vi "Update Position.vi"(11 "Motion in":refnum<class "Motion.lvclass">) -> (3 "Motion out":refnum<class "Motion.lvclass">)   [LabVIEW 2021, in "Motion.lvclass"]
uses:
  Motion.lvclass
  Motion.lvclass/Motion.ctl
  Re-use Libraries/Vector 2D/Vector 2D.lvclass
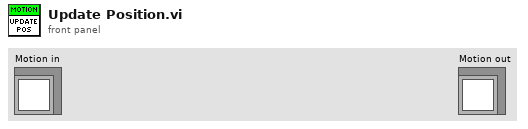
[diagram p1: front panel]
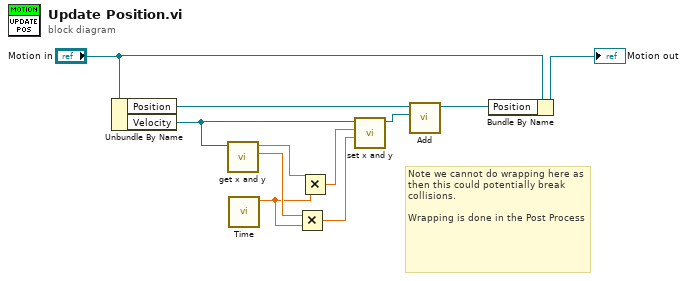
[diagram p0: block diagram]
diagram:
  # "Note we cannot do wrapping here as then this could potentially break collisions.\n\nWrapping is done in the Post Process"
  n1 = Unbundle By Name("Motion in") -> ("Position"=w11:refnum<class "Vector 2D.lvclass">, "Velocity"=w6:refnum<class "Vector 2D.lvclass">)
  n2 = call "get x and y.vi"("Vector 2D in"=w6) -> ("y"=w3:sgl, "x"=w5:sgl)  [unwired: 9 in]
  n3 = call "Time.vi"() -> ("Delta Time [s]"=w1:sgl)  [unwired: 10 in, 1 out]
  n4 = Multiply(x=w3, y=w1) -> (x*y=w2:sgl)
  n5 = Multiply(x=w5, y=w1) -> (x*y=w4:sgl)
  n6 = call "set x and y.vi"("y"=w2, "x"=w4, "Vector 2D in"=w6) -> ("Vector 2D out"=w8:refnum<class "Vector 2D.lvclass">)  [unwired: 8 in]
  n7 = call "Add.vi"("B"=w8, "A"=w11) -> ("A+B"=w7:refnum<class "Vector 2D.lvclass">)  [unwired: 9 in]
  n8 = Bundle By Name(cluster="Motion in", "Position"=w7) -> (→"Motion out":refnum<class "Motion.lvclass">)
